vi "Get Configuration Cluster.vi"(8 "error in (no error)":errorcluster, 11 "Transfer Configuration in":refnum<class "Transfer Configuration.lvclass">) -> (0 "error out":errorcluster, 2 "transfer configuration":T1={"core"={"name"="Transfer"}, "component settings"=[], "channels"=[]} {"channels"."core"."string offset" format="%d bytes"}, 3 "Transfer Configuration out":refnum<class "Transfer Configuration.lvclass">)   [LabVIEW 2020, in "DSF Core.lvlib" / "Transfer Configuration.lvclass"]
uses:
  Transfer Configuration.lvclass
  C:/Users/nitest/Desktop/Git/niveristand-data-sharing-framework-custom-device/Source/Core/Classes/Configuration/Core/Core Configuration.lvclass
  Typedefs/DSF Engine Transfer Configuration.ctl
  Typedefs/Core Transfer Configuration.ctl
  Typedefs/DSF Settings Info.ctl
  Typedefs/DSF Engine Channel Configuration.ctl
  Typedefs/Core Channel Configuration.ctl
  Typedefs/DSF Data Type.ctl
  Transfer Configuration.lvclass/Transfer Configuration.ctl
  DSF Core.lvlib
  Core Configuration.lvclass
  Channel/Channel Configuration.lvclass
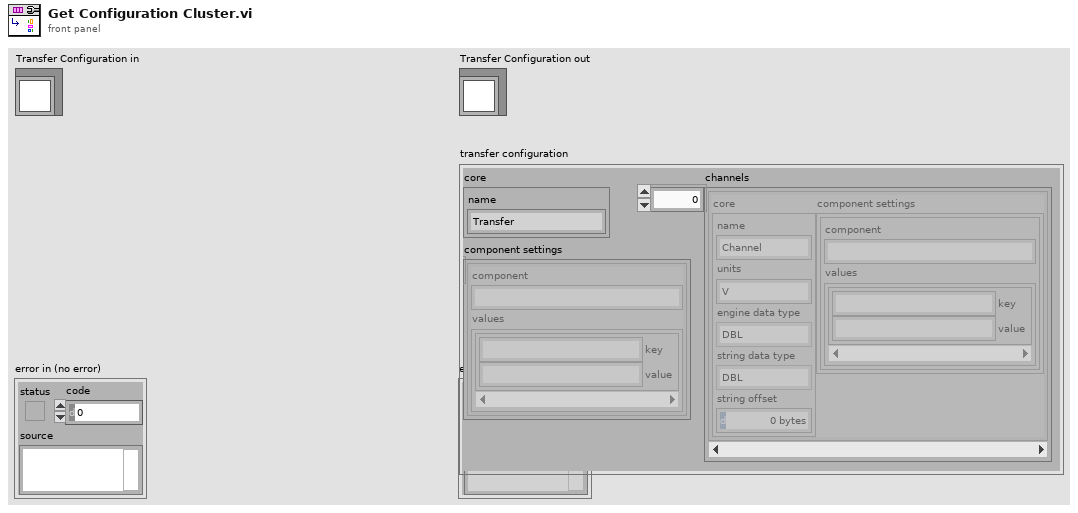
[diagram p1: front panel]
types:
  T1 = typedef "DSF Core.lvlib/DSF Engine Transfer Configuration.ctl" = cluster{"core":T2, "component settings":T3[], "channels":T4[]}
  T2 = typedef "DSF Core.lvlib/Transfer Configuration.lvclass/Core Transfer Configuration.ctl" = cluster{"name":string}
  T3 = typedef "DSF Core.lvlib/DSF Settings Info.ctl" = cluster{"component":string, "values":cluster{"key":string, "value":string}[]}
  T4 = typedef "DSF Core.lvlib/DSF Engine Channel Configuration.ctl" = cluster{"core":T5, "component settings":T3[]}
  T5 = typedef "DSF Core.lvlib/Channel Configuration.lvclass/Core Channel Configuration.ctl" = cluster{"name":string, "units":string, "engine data type":T6, "string data type":T6, "string offset":u64}
  T6 = typedef "DSF Core.lvlib/DSF Data Type.ctl" = enum8{"Bool", "SGL", "DBL", "I8", "I16", "I32", "I64", "U8", "U16", "U32", "U64"}
  T7 = typedef "DSF Core.lvlib/Transfer Configuration.lvclass/Channel Configuration.ctl" = cluster{"configuration":T5, "component settings":T3[]}
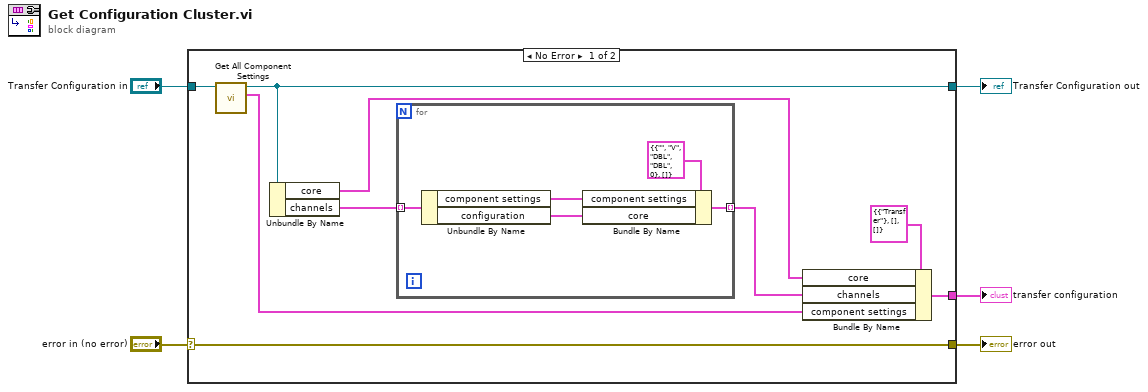
[diagram p0: block diagram]
diagram:
  n1 = case shown="No Error" "error in (no error)" {
    selector: "error in (no error)" -> [w6 w21]
    tunnel: [w6 w21] -> w4
    tunnel: [w7 w20] -> w2
    tunnel: "Transfer Configuration in" -> [w12 w20]
    tunnel: [w13 _] -> w1
    frame No Error {
      n2 = call "Get All Component Settings.vi"("Runtime Configuration in"=w12) -> ("component settings"=w9:T3[], "Runtime Configuration out"=w7:refnum<class "Transfer Configuration.lvclass">)  [unwired: 8 in, 1 out]
      n3 = Unbundle By Name(w7) -> ("core"=w8:T2, "channels"=w11:T7[])
      n4 = for {
        tunnel: w11 -> [w19] mode=indexing
        tunnel: [w16] -> w10 mode=indexing
        n5 = Unbundle By Name(w19) -> ("component settings"=w17:T3[], "configuration"=w15:T5)
        n6 = Bundle By Name(cluster=T4 {"core"={"name"="", "units"="V", "engine data type"=enum."DBL", "string data type"=enum."DBL", "string offset"=0}, "component settings"=[]} ("channels"), "component settings"=w17, "core"=w15) -> (w16:T4)
      }
      n7 = Bundle By Name(cluster=T1 {"core"={"name"="Transfer"}, "component settings"=[], "channels"=[]} ("transfer configuration"), "core"=w8, "channels"=w10, "component settings"=w9) -> (w13:T1)
    }
    frame Error {
    }
  }
  "error out" <- w4
  "Transfer Configuration out" <- w2
  "transfer configuration" <- w1
